vi "rytimer_palette.vi"   [LabVIEW 2017]
uses:
  enqueue.ctl
  rytimer.lvclass/rytimer.ctl
  rytimer.lvclass
types:
  T1 = typedef "rytimer.lvclass/enqueue.ctl" = enum8{"back", "front", "back_if_absent", "front_if_absent"}
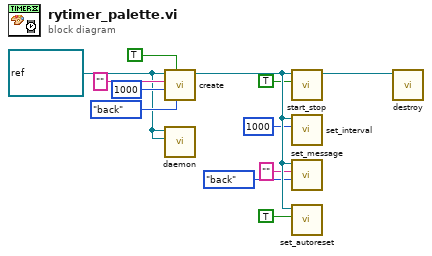
[diagram p0: block diagram]
diagram:
  w1 = refnum<queue> refnum ("destination queue")
  n1 = call "create.vi"("enqueue (back)"=enqueue."back", "auto-reset? (T)"=TRUE, "interval (1000 ms)"=u32 1000, "message (\"\"=Ignore)"="" ("message (\"\"=Ignore)"), "destination queue"=w1) -> ("timer"=w11:refnum<class "rytimer.lvclass">)  [unwired: 5 in, 1 out]
  n2 = call "daemon.vi"("queue"=w1, "timer"=w1) -> ()  [unwired: 10 in]
  n3 = call "start_stop.vi"("start? (T)"=TRUE, "timer in"=w11) -> ("timer out"=w12:refnum<class "rytimer.lvclass">)  [unwired: 8 in, 1 out]
  n4 = call "set_interval.vi"("interval (1000 ms)"=u32 1000, "timer in"=w11) -> ()  [unwired: 8 in, 2 out]
  n5 = call "set_message.vi"("enqueue (back)"=enqueue."back", "message"="", "timer in"=w11) -> ()  [unwired: 7 in, 2 out]
  n6 = call "set_autoreset.vi"("auto-reset? (T)"=TRUE, "timer in"=w11) -> ()  [unwired: 8 in, 2 out]
  n7 = call "destroy.vi"("timer"=w12) -> ()  [unwired: 10 in, 1 out]
